vi "testing.vi"() -> ()   [LabVIEW 2017]
panel:
  out "x+y":dbl
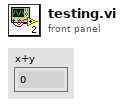
[diagram p1: front panel]
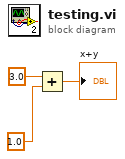
[diagram p0: block diagram]
diagram:
  n1 = Add(x=3.0, y=1.0) -> (x+y=→"x+y":dbl)
